vi "Read dt.vi"(8 "error in (no error)":errorcluster, 11 "CRDS in":refnum<class "CRDS.lvclass">) -> (0 "error out":errorcluster, 2 "dt":sgl, 3 "CRDS out":refnum<class "CRDS.lvclass">)   [LabVIEW 2011, in "CRDS.lvclass"]
uses:
  CRDS.lvclass
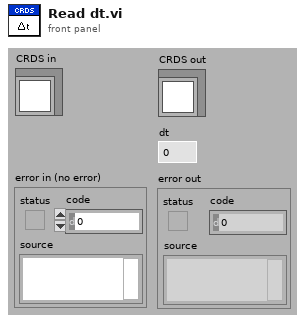
[diagram p1: front panel]
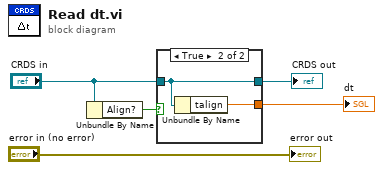
[diagram p0: block diagram]
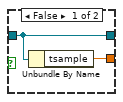
[diagram p2: hidden frame]
diagram:
  n1 = Unbundle By Name("CRDS in") -> ("Align?"=w2:bool)
  n2 = case shown="True" w2 {
    tunnel: "CRDS in" -> [w7 w9]
    tunnel: [w7 w9] -> w3
    tunnel: [w6 w8] -> w1
    frame False {
      n3 = Unbundle By Name(w7) -> ("tsample"=w6:sgl)
    }
    frame True {
      n4 = Unbundle By Name(w9) -> ("talign"=w8:sgl)
    }
  }
  "CRDS out" <- w3
  "dt" <- w1
  "error out" <- "error in (no error)"
